vi "MPM_Information.vi"(0 ".NET Reference in":refnum<k24>, 11 "error in (no error)":errorcluster) -> (1 "ModuleFW":string[](array[string]), 3 "ProductName":string, 4 "Reference out":refnum<k24>, 6 "FWversion":string, 8 "SerialNumber":string, 10 "NumberofModule":i32, 12 "ModuelSerial":string[](array[string]), 14 "ModuleType":string[](array[string]), 15 "error out":errorcluster)   [LabVIEW 2017]
uses:
  C:/Users/Ssantec_Test/Documents/Instrument_DLL_Sample_Labview_20220902_Ver1.2.2/DLL/x86/InstrumentDLL.dll
  DLL/x86/InstrumentDLL.dll
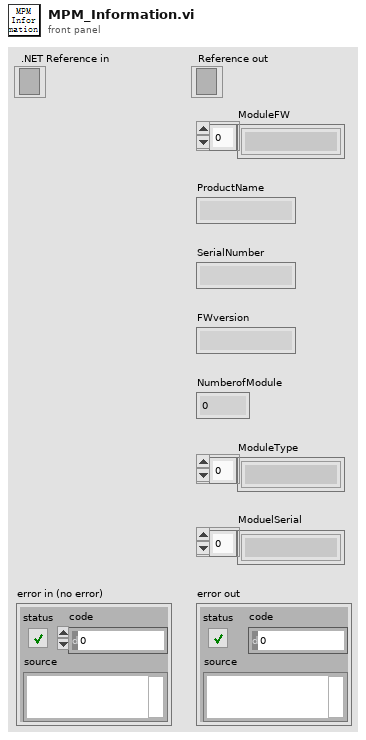
[diagram p1: front panel]
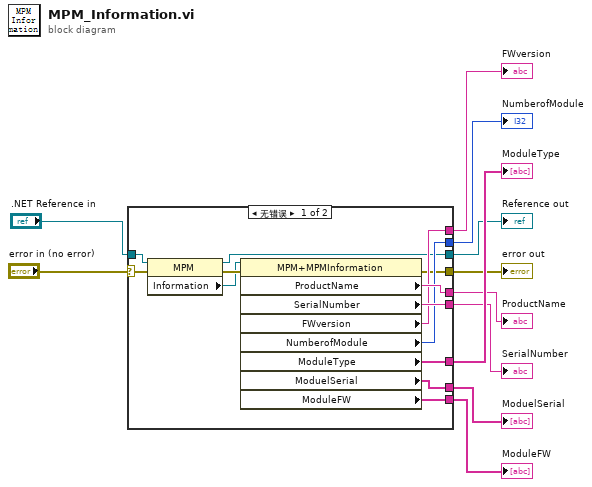
[diagram p0: block diagram]
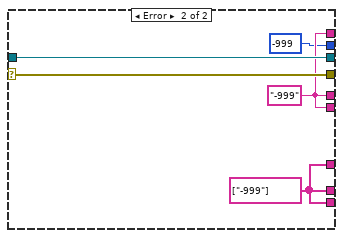
[diagram p2: hidden frame]
diagram:
  n1 = case shown="无错误" "error in (no error)" {
    selector: "error in (no error)" -> [w15 w28]
    tunnel: [w24 w27] -> w11
    tunnel: [w23 w27] -> w10
    tunnel: [w22 w27] -> w9
    tunnel: [w21 w26] -> w8
    tunnel: [w20 w26] -> w7
    tunnel: [w19 w26] -> w6
    tunnel: [w18 -999 ("NumberofModule")] -> w5
    tunnel: ".NET Reference in" -> [w16 w29]
    tunnel: [w12 w29] -> w1
    tunnel: [w17 w28] -> w4
    frame No Error {
      n2 = property on="属性节点" class="MPM"(reference=w16, error in=w15) -> (reference out=w12:refnum<k24>, error out=w14:errorcluster, "Information"=w13:refnum<k24>)
      n3 = property on="属性节点" class="MPM+MPMInformation"(reference=w13, error in=w14) -> (error out=w17:errorcluster, "ProductName"=w21:string, "SerialNumber"=w20:string, "FWversion"=w19:string, "NumberofModule"=w18:i32, "ModuleType"=w24:string[], "ModuelSerial"=w22:string[], "ModuleFW"=w23:string[])  [unwired: 1 out]
    }
    frame Error {
      w26 = "-999" ("FWversion")
      w27 = string[] ["-999"] ("ModuleFW")
    }
  }
  "ModuleType" <- w11
  "ModuleFW" <- w10
  "ModuelSerial" <- w9
  "ProductName" <- w8
  "SerialNumber" <- w7
  "FWversion" <- w6
  "NumberofModule" <- w5
  "error out" <- w4
  "Reference out" <- w1
